vi "Write to Serial Port.vi"(6 "Tx String":refnum<vi>, 8 "error in (no error)":errorcluster, 9 "Transmit?":bool, 10 "Clear after send?":bool, 11 "VISA refnum in":refnum<visa-resource-name>) -> (0 "error out":errorcluster, 3 "VISA refnum out":refnum<visa-resource-name>)   [LabVIEW 2024]
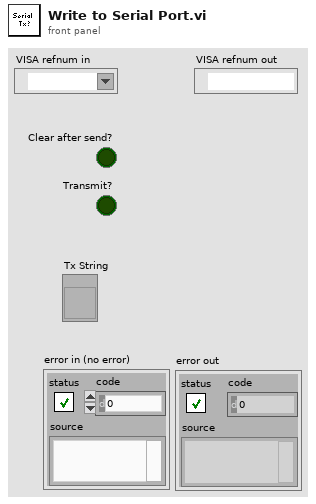
[diagram p1: front panel]
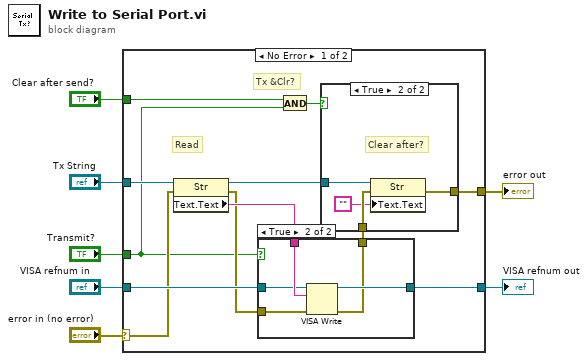
[diagram p0: block diagram]
diagram:
  n1 = case shown="No Error" "error in (no error)" {
    selector: "error in (no error)" -> [w9 w32]
    tunnel: "Tx String" -> [w19 _]
    tunnel: "VISA refnum in" -> [w17 w33]
    tunnel: [w13 w32] -> w4
    tunnel: [w16 w33] -> w3
    tunnel: "Clear after send?" -> [w11 _]
    tunnel: "Transmit?" -> [w8 _]
    frame No Error {
      # "Tx &Clr?"
      # "Read"
      n2 = property class="Str"(reference=w19, error in=w9) -> (reference out=w15:refnum<vi>, error out=w12:errorcluster, "Text.Text"=w18:string)
      n3 = case shown="True" w8 {
        tunnel: w18 -> [_ w26]
        tunnel: w17 -> [w21 w25]
        tunnel: [w21 w24] -> w16
        tunnel: [w20 w23] -> w14
        tunnel: w12 -> [w20 w22]
        frame False {
        }
        frame True {
          n4 = VISA Write(VISA resource name=w25, write buffer=w26, error in (no error)=w22) -> (VISA resource name out=w24:refnum<visa-resource-name>, error out=w23:errorcluster)  [unwired: 1 out]
        }
      }
      n5 = And(x=w11, y=w8) -> (x .and. y?=w10:bool)
      n6 = case shown="True" w10 {
        tunnel: w15 -> [_ w31]
        tunnel: w14 -> [w27 w30]
        tunnel: [w27 w29] -> w13
        frame False {
        }
        frame True {
          # "Clear after?"
          n7 = property class="Str"(reference=w31, error in=w30, "Text.Text"="") -> (error out=w29:errorcluster)  [unwired: 1 out]
        }
      }
    }
    frame Error {
    }
  }
  "VISA refnum out" <- w3
  "error out" <- w4
